vi "DDS9959 Frequency String.vi"(10 "Clock Frequency (MHz)":dbl, 11 "Set Frequency (MHz)":dbl) -> (3 "String":string)   [LabVIEW 2012]
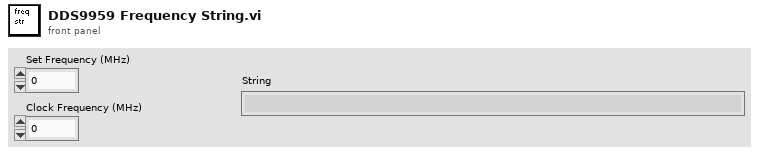
[diagram p1: front panel]
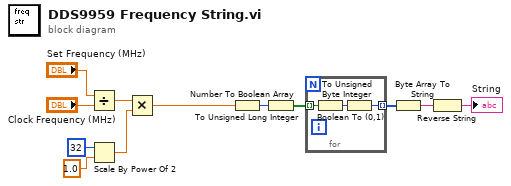
[diagram p0: block diagram]
diagram:
  n1 = Divide(x="Set Frequency (MHz)", y="Clock Frequency (MHz)") -> (x/y=w10:dbl)
  n2 = Scale By Power Of 2(n=32, x=1.0) -> (x*2^n=w7:dbl)
  n3 = Multiply(x=w10, y=w7) -> (x*y=w1:dbl)
  n4 = To Unsigned Long Integer(number=w1) -> (unsigned 32bit integer=w3:u32)
  n5 = Number To Boolean Array(number=w3) -> (Boolean array=w6:bool[])
  n6 = for {
    tunnel: w6 -> [w15] mode=indexing
    tunnel: [w13] -> w5 mode=indexing
    n7 = Boolean To (0,1)(Boolean=w15) -> (0, 1=w14:i16)
    n8 = To Unsigned Byte Integer(number=w14) -> (unsigned 8bit integer=w13:u8)
  }
  n9 = Byte Array To String(unsigned byte array=w5) -> (string=w4:string)
  n10 = Reverse String(1:w4) -> (0:→"String":string)
